vi "Remove Extension from Str.vi"(8 "error in (no error)":errorcluster, 11 "Name":string) -> (0 "error out":errorcluster, 3 "Name Without Extension":string)   [LabVIEW 2020, in "ADAS_IO_Template_MDO.lvclass"]
uses:
  ADAS_IO_Template_MDO.lvclass
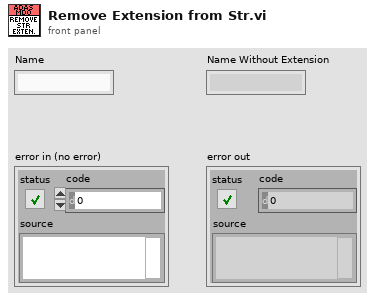
[diagram p1: front panel]
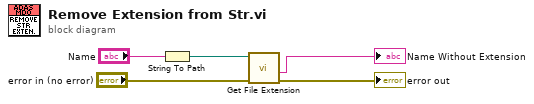
[diagram p0: block diagram]
diagram:
  n1 = String To Path(string="Name") -> (path=w4:path)
  n2 = call <vilib>:"Get File Extension.vi"("error in (no error)"="error in (no error)", "file"=w4) -> ("error out"=→"error out":errorcluster, "filename without extension"=→"Name Without Extension":string)  [unwired: 5 in, 3 out]
